vi "S8300E_Chk_DIMM_Quality.vi"() -> ()   [LabVIEW 2011]
uses:
  <vilib>/Instr/_visa.llb/VISA Set IO Buffer Mask.ctl
panel:
  out "FinalLOG1":string
  out "log1":string
  out "DIMM":T1
  out "LOG":string
  out "VISA6":refnum<visa-resource-name>
  out "BEGIN TIME":u32
  out "進行狀況":string
  # "Error Code:DIMM"
  # "S8300E Screen out Defect DIMM Modules"
  # "2015-8-21"
  # "Need S8300E Test Board + S8300E MB\n1.Check 2 DIMM Modules\nConcept: When DIMM Modules go abnoraml, CPLD will set LED12 during bootup periodof time.\n如果系統回報NG ,請把兩條DIMM Modules 貼NG Label."
  # "PC COM6 Baud  115200 -->Test Board UART"
  # "Test Board\nBP_PIC_BRD_IN_N"
  # "S8300E MB\nCPLD_PLTRST_LED_N"
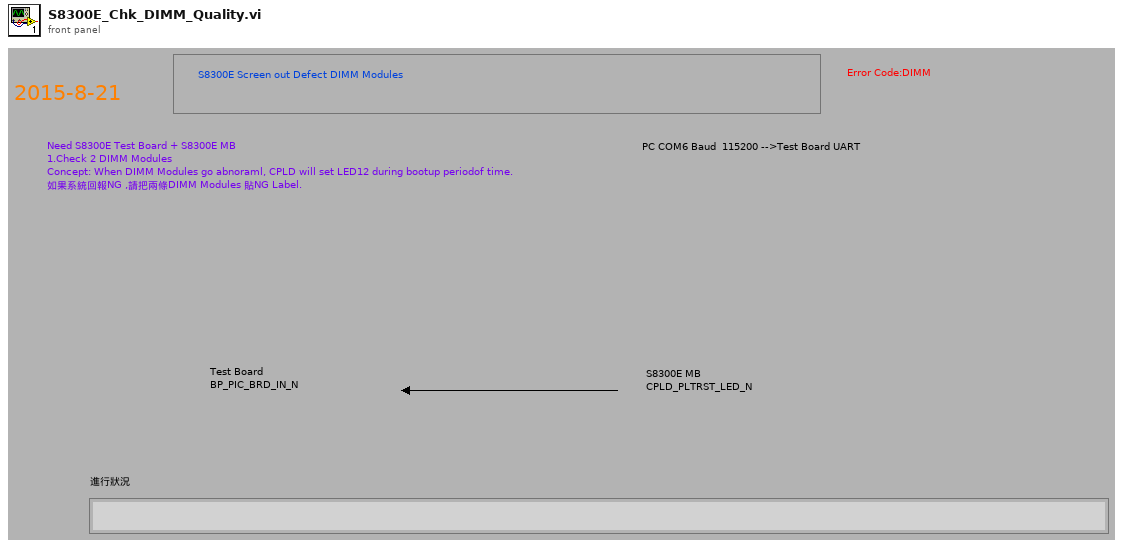
[diagram p1: front panel]
types:
  T1 = cluster{string, "Find this String":string, "Find this String":string}
  T2 = typedef "VISA Set IO Buffer Mask.ctl" = u16
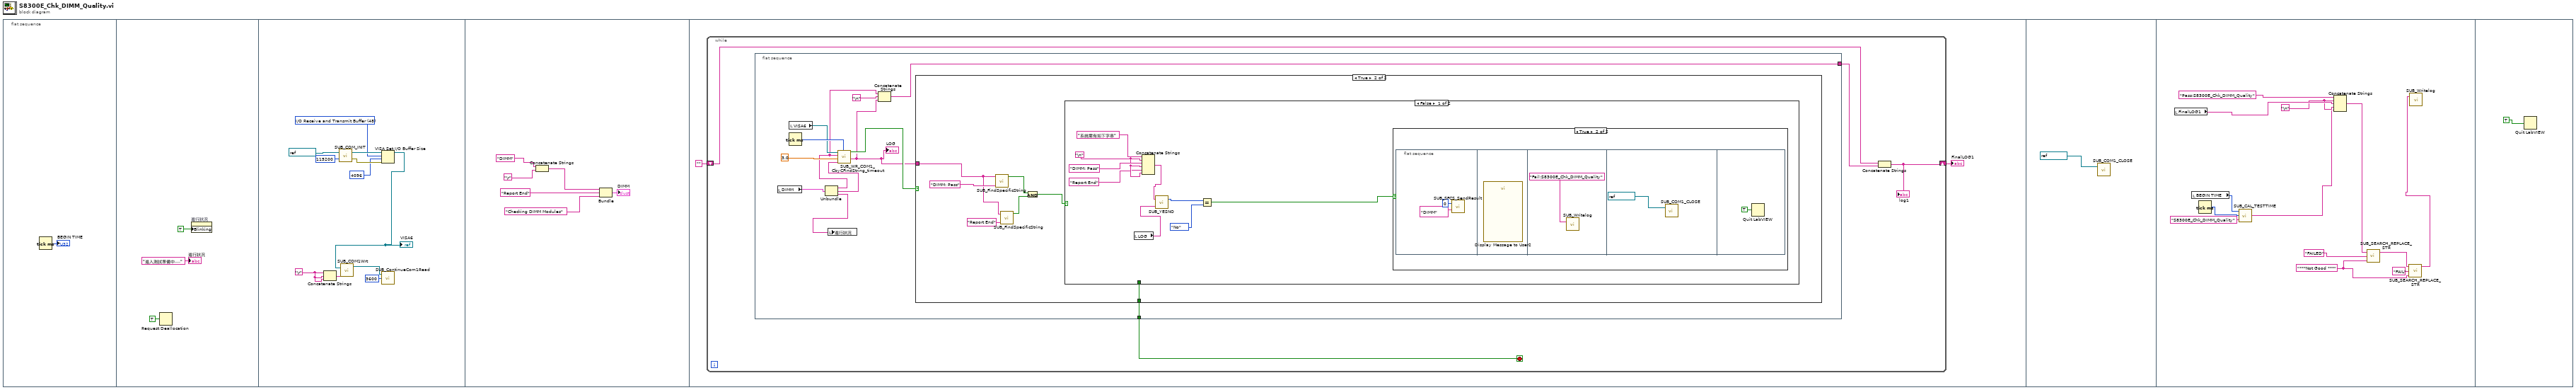
[diagram p0: block diagram]
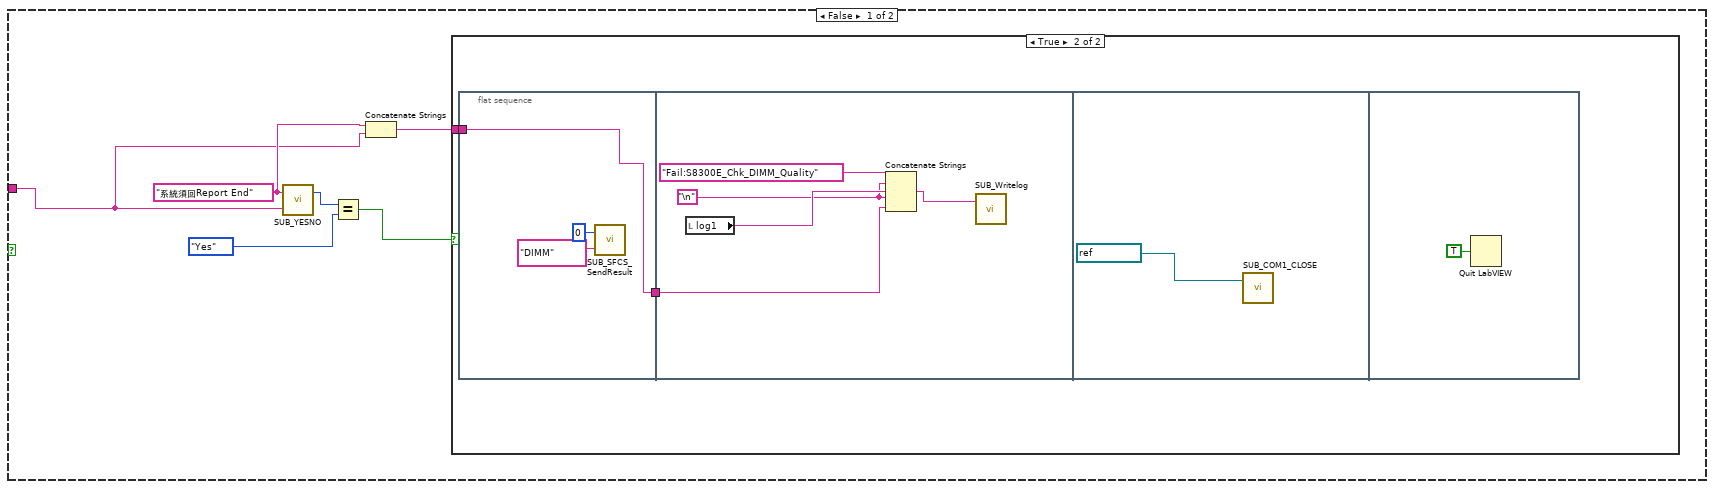
[diagram p2: hidden frame]
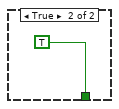
[diagram p5: hidden frame]
diagram:
  n1 = flat-sequence {
    frame #0 {
      n2 = Tick Count (ms)() -> (millisecond timer value=→"BEGIN TIME":u32)
    }
    frame #1 {
      n3 = Request Deallocation(TRUE ("flag")) -> ()
      n4 = property on="進行狀況" class="Str"("Blinking"=TRUE) -> ()  [unwired: 2 in, 2 out]
      "進行狀況" <- "進入測試準備中...." ("進行狀況")
    }
    frame #2 {
      w5 = T2 48 items=["I/O Receive Buffer"=16, "I/O Transmit Buffer"=32, "I/O Receive and Transmit Buffer"=48] ("Mask")
      w14 = "\r"
      n5 = Concatenate Strings(w14, w14, w14) -> (w13:string)
      n6 = call "SUB_COM_INIT.vi"("baud rate (9600)"=u32 115200, "VISA resource name"=refnum<visa-resource-name> "COM6") -> ("error out"=w8:errorcluster, "VISA resource name out"=w9:refnum<visa-resource-name>)
      n7 = VISA Set I/O Buffer Size(VISA resource name=w9, mask (16)=w5, size (4096)=u32 4096, error in (no error)=w8) -> (VISA resource name out=w7:refnum<visa-resource-name>)  [unwired: 1 out]
      "VISA6" <- w7
      n8 = call "SUB_COM1Wrt.vi"("VISA resource name"=w7, "write buffer"=w13) -> ("duplicate VISA resource name"=w12:refnum<visa-resource-name>)  [unwired: 1 in, 1 out]
      n9 = call "SUB_ContinueCom1Read.vi"("Numeric"=3600, "duplicate VISA resource name 2"=w12) -> ()  [unwired: 1 in, 3 out]
    }
    frame #3 {
      n10 = Concatenate Strings("DIMM" ("Find this String"), "\r") -> (w17:string)
      n11 = Bundle(w17, "Find this String"="Report End", "Find this String"="Checking DIMM Modules") -> (→"DIMM":T1)  [unwired: 1 in]
    }
    frame #4 {
      n12 = while {
        shift-right: [w26] -> w22
        shift-left: "" -> [w25]
        stop <- w27 stop-if-true
        n13 = flat-sequence {
          tunnel: [w32] -> w27
          tunnel: [w28] -> w24
          frame #0 {
            n14 = local read "DIMM"() -> (w36:T1)
            n15 = Tick Count (ms)() -> (millisecond timer value=w39:u32)
            n16 = local read "VISA6"() -> (w37:refnum<visa-resource-name>)
            n17 = Unbundle(w36) -> (w31:string, "Find this String"=w35:string, "Find this String"=w34:string)
            n18 = local write "進行狀況"(w34) -> ()
            n19 = call "SUB_WR_COM1_CbyCFindString_timeout.vi"("Begin time"=w39, "Find this String"=w35, "Timeout Seccond"=3.0, "cmd string"=w31, "duplicate VISA resource name 2"=w37) -> ("Output String"=w29:string, "Found String"=w33:bool)  [unwired: 2 out]
            "LOG" <- w29
            n20 = Concatenate Strings(w31, "\n", w29) -> (w28:string)
            n21 = case shown="True" w33 {
              tunnel: w29 -> [w41 w63]
              tunnel: [_ w59] -> w32
              frame False {
                w42 = "系統須回Report End" ("Status")
                n22 = call "SUB_YESNO.vi"("Debug View"=w41, "Status"=w42) -> ("yes/no"=w45:enum32{"No Selection", "Yes", "No", "None"})  [unwired: 1 in]
                n23 = Equal?(x=w45, y=enum32{"No Selection", "Yes", "No", "None"}."Yes") -> (x = y?=w43:bool)
                n24 = Concatenate Strings(w42, w41) -> (w40:string)
                n25 = case shown="True" w43 {
                  tunnel: w40 -> [_ w46]
                  frame False {
                  }
                  frame True {
                    n26 = flat-sequence {
                      tunnel: [w48] -> w47
                      tunnel: w46 -> [w48]
                      tunnel: w47 -> [w51]
                      frame #0 {
                        n27 = call "SUB_SFCS_SendResult.vi"("ErrorCode"="DIMM", "PASS_Fail (1/0)"=i8 0) -> ()  [unwired: 1 out]
                      }
                      frame #1 {
                        w52 = "\n"
                        n28 = local read "log1"() -> (w54:string)
                        n29 = Concatenate Strings("Fail:S8300E_Chk_DIMM_Quality" ("Pass/Fail"), w52, w54, w52, w51) -> (w53:string)
                        n30 = call "SUB_Writelog.vi"("Pass/Fail"=w53) -> ()  [unwired: 2 in]
                      }
                      frame #2 {
                        n31 = call "SUB_COM1_CLOSE.vi"("VISA resource name"=refnum<visa-resource-name> "COM6") -> ()  [unwired: 3 in]
                      }
                      frame #3 {
                        n32 = Quit LabVIEW(quit? (T)=TRUE) -> ()
                      }
                    }
                  }
                }
              }
              frame True {
                n33 = call "SUB_FindSpecificString.vi"("Find this String"="DIMM: Pass", "String data"=w63) -> ("Found"=w62:bool)  [unwired: 2 in, 1 out]
                n34 = call "SUB_FindSpecificString.vi"("Find this String"="Report End", "String data"=w63) -> ("Found"=w61:bool)  [unwired: 2 in, 1 out]
                n35 = And(x=w62, y=w61) -> (x .and. y?=w60:bool)
                n36 = case shown="False" w60 {
                  tunnel: [_ TRUE] -> w59
                  frame False {
                    w70 = "\n"
                    n37 = local read "LOG"() -> (w73:string)
                    n38 = Concatenate Strings("系統需有如下字串" ("string"), w70, "DIMM: Pass" ("Find this String"), w70, "Report End" ("Find this String"), w70) -> (w69:string)
                    n39 = call "SUB_YESNO.vi"("Debug View"=w73, "Status"=w69) -> ("yes/no"=w68:enum32{"No Selection", "Yes", "No", "None"})  [unwired: 1 in]
                    n40 = Equal?(x=w68, y=enum32{"No Selection", "Yes", "No", "None"}."No") -> (x = y?=w66:bool)
                    n41 = case shown="True" w66 {
                      frame False {
                      }
                      frame True {
                        n42 = flat-sequence {
                          frame #0 {
                            n43 = call "SUB_SFCS_SendResult.vi"("ErrorCode"="DIMM", "PASS_Fail (1/0)"=i8 0) -> ()  [unwired: 1 out]
                          }
                          frame #1 {
                            n44 = call "Display Message to User2"() -> ()  [unwired: 10 in, 2 out]
                          }
                          frame #2 {
                            n45 = call "SUB_Writelog.vi"("Pass/Fail"="Fail:S8300E_Chk_DIMM_Quality") -> ()  [unwired: 2 in]
                          }
                          frame #3 {
                            n46 = call "SUB_COM1_CLOSE.vi"("VISA resource name"=refnum<visa-resource-name> "COM6") -> ()  [unwired: 3 in]
                          }
                          frame #4 {
                            n47 = Quit LabVIEW(quit? (T)=TRUE) -> ()
                          }
                        }
                      }
                    }
                  }
                  frame True {
                  }
                }
              }
            }
          }
        }
        n48 = Concatenate Strings(w25, w24) -> (w26:string)
        "log1" <- w26
      }
      "FinalLOG1" <- w22
    }
    frame #5 {
      n49 = call "SUB_COM1_CLOSE.vi"("VISA resource name"=refnum<visa-resource-name> "COM6") -> ()  [unwired: 3 in]
    }
    frame #6 {
      w85 = "***Not Good ***" ("replace string (\"\")")
      w82 = "\n"
      n50 = local read "FinalLOG1"() -> (w89:string)
      n51 = local read "BEGIN TIME"() -> (w92:u32)
      n52 = Tick Count (ms)() -> (millisecond timer value=w91:u32)
      n53 = call "SUB_CAL_TESTTIME.vi"("Test Item name"="S8300E_Chk_DIMM_Quality", "Stop tick time"=w91, "Start tick time"=w92) -> ("Test Time output"=w81:string)  [unwired: 2 in]
      n54 = Concatenate Strings("Pass:S8300E_Chk_DIMM_Quality", w82, w89, w82, w81) -> (w83:string)
      n55 = call "SUB_SEARCH_REPLACE_STR.vi"("replace string (\"\")"=w85, "search string"="FAILED", "input string"=w83) -> ("result string"=w87:string)  [unwired: 2 in]
      n56 = call "SUB_SEARCH_REPLACE_STR.vi"("replace string (\"\")"=w85, "search string"="FAIL", "input string"=w87) -> ("result string"=w84:string)  [unwired: 2 in]
      n57 = call "SUB_Writelog.vi"("Pass/Fail"=w84) -> ()  [unwired: 2 in]
    }
    frame #7 {
      n58 = Quit LabVIEW(quit? (T)=TRUE ("stop? (T)")) -> ()
    }
  }
